vi "Update String Value.vi"(9 "Value":string, 10 "Tree Tag":string, 11 "Settings In":T1) -> (3 "Settings Out":T1)   [LabVIEW 2020, in "Sequencer with Output Values.lvlib" / "Sequencer with Output Values.lvclass"]
uses:
  Sequencer with Output Values.lvclass
  Params.ctl
  Step Settings.ctl
  Global Tree Data.vi
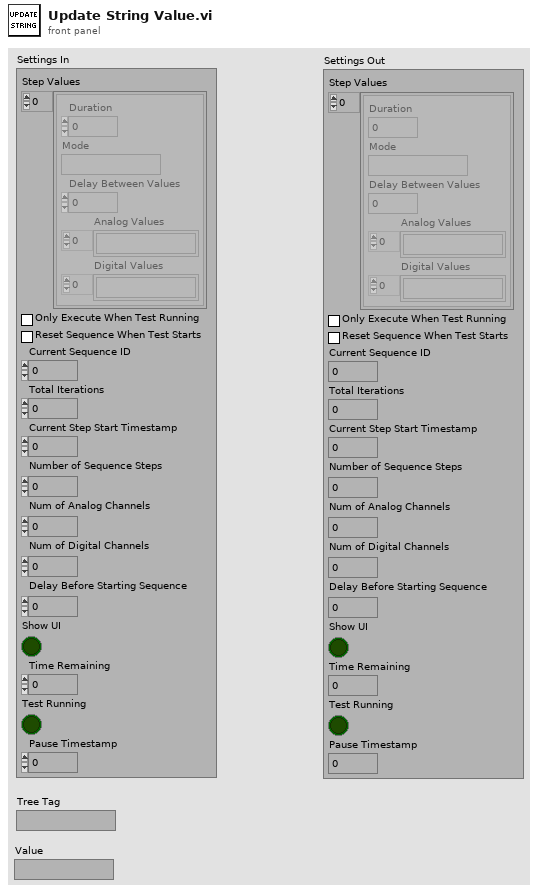
[diagram p1: front panel]
types:
  T1 = typedef "Sequencer with Output Values.lvlib/Sequencer with Output Values.lvclass/Params.ctl" = cluster{"Step Values":T2[], "Only Execute When Test Running":bool, "Reset Sequence When Test Starts":bool, "Current Sequence ID":u32, "Total Iterations":u32, "Current Step Start Timestamp":dbl, "Number of Sequence Steps":i32, "Num of Analog Channels":i32, "Num of Digital Channels":i32, "Delay Before Starting Sequence":dbl, "Show UI":bool, "Time Remaining":dbl, "Test Running":bool, "Pause Timestamp":dbl}
  T2 = typedef "Sequencer with Output Values.lvlib/Sequencer with Output Values.lvclass/Step Settings.ctl" = cluster{"Duration":dbl, "Mode":string, "Delay Between Values":dbl, "Analog Values":string[], "Digital Values":string[]}
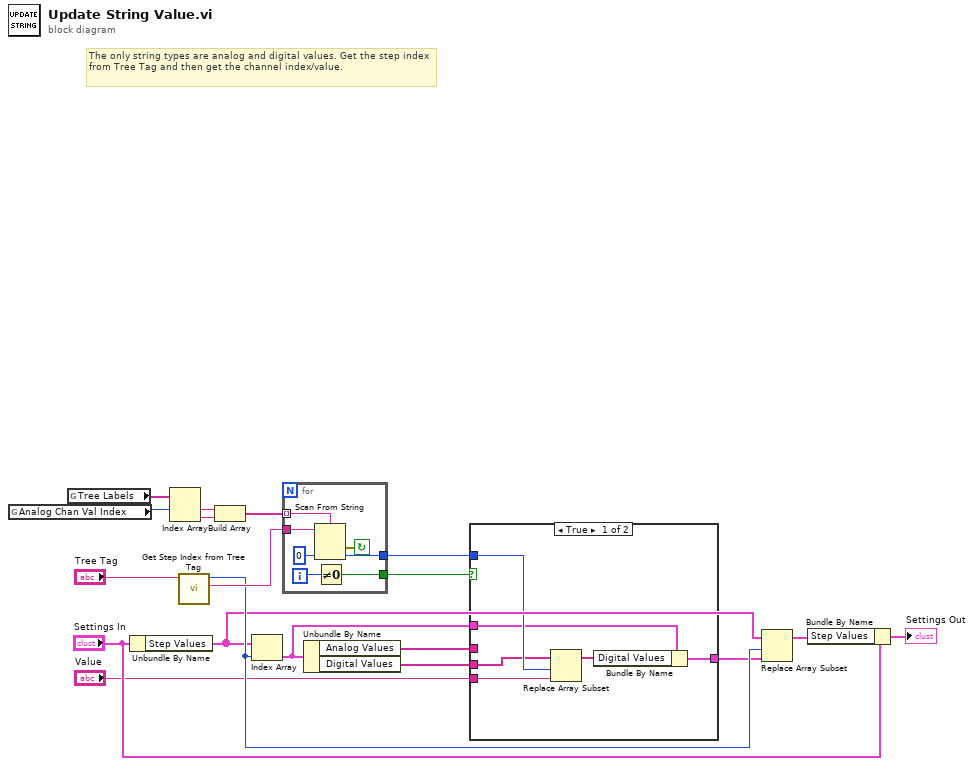
[diagram p0: block diagram]
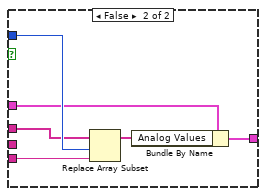
[diagram p2: hidden frame]
diagram:
  # "The only string types are analog and digital values. Get the step index from Tree Tag and then get the channel index/value."
  n1 = global read "Global Tree Data.vi" "Analog Chan Val Index"() -> (w17:i32)
  n2 = global read "Global Tree Data.vi" "Tree Labels"() -> (w18:string[])
  n3 = Unbundle By Name("Settings In") -> ("Step Values"=w6:T2[])
  n4 = Index Array(array=w18, index #1=w17) -> (element #1=w15:string, element #2=w14:string)  [unwired: 1 in]
  n5 = call "Get Step Index from Tree Tag.vi"("Tree Tag"="Tree Tag") -> ("Step Param String"=w16:string, "Step Index"=w7:i32)  [unwired: 9 in]
  n6 = Build Array(w15, w14) -> (w13:string[])
  n7 = Index Array(array=w6, index=w7) -> (element=w10:T2)
  n8 = for {
    tunnel: w16 -> [w25]
    tunnel: w13 -> [w24] mode=indexing
    tunnel: [w21] -> w11
    tunnel: [w20] -> w12
    i -> [w22]
    stop <- w23 continue-if-true
    n9 = Scan From String(format string=w24, input string=w25, default 1=0) -> (error out=w23:errorcluster, output 1=w20:i32)  [unwired: 2 in, 2 out]
    n10 = Not Equal To 0?(x=w22) -> (x != 0?=w21:bool)
  }
  n11 = Unbundle By Name(w10) -> ("Analog Values"=w9:string[], "Digital Values"=w8:string[])
  n12 = case shown="True" w11 {
    tunnel: w12 -> [w32 w38]
    tunnel: "Value" -> [w31 w37]
    tunnel: w10 -> [w30 w36]
    tunnel: w9 -> [_ w33]
    tunnel: w8 -> [w29 _]
    tunnel: [w27 w34] -> w5
    frame True {
      n13 = Replace Array Subset(array=w29, new element=w31, index=w32) -> (w28:string[])
      n14 = Bundle By Name(cluster=w30, "Digital Values"=w28) -> (w27:T2)
    }
    frame False {
      n15 = Replace Array Subset(array=w33, new element=w37, index=w38) -> (w35:string[])
      n16 = Bundle By Name(cluster=w36, "Analog Values"=w35) -> (w34:T2)
    }
  }
  n17 = Replace Array Subset(array=w6, new element=w5, index=w7) -> (w3:T2[])
  n18 = Bundle By Name(cluster="Settings In", "Step Values"=w3) -> (→"Settings Out":T1)
